vi "VI Tree - string__ogtk.vi"   [LabVIEW 2009]
uses:
  Trim Whitespace (String)__ogtk.vi
  Convert EOLs (String)__ogtk.vi
  To Camel Case (String)__ogtk.vi
  To Proper Case (String)__ogtk.vi
  To Proper Case (String Array)__ogtk.vi
  Trim Whitespace (String Array)__ogtk.vi
  To Camel Case (String Array)__ogtk.vi
  Convert EOLs (String Array)__ogtk.vi
panel:
  # "[OpenG VI Tags] ***Do Not Remove***"
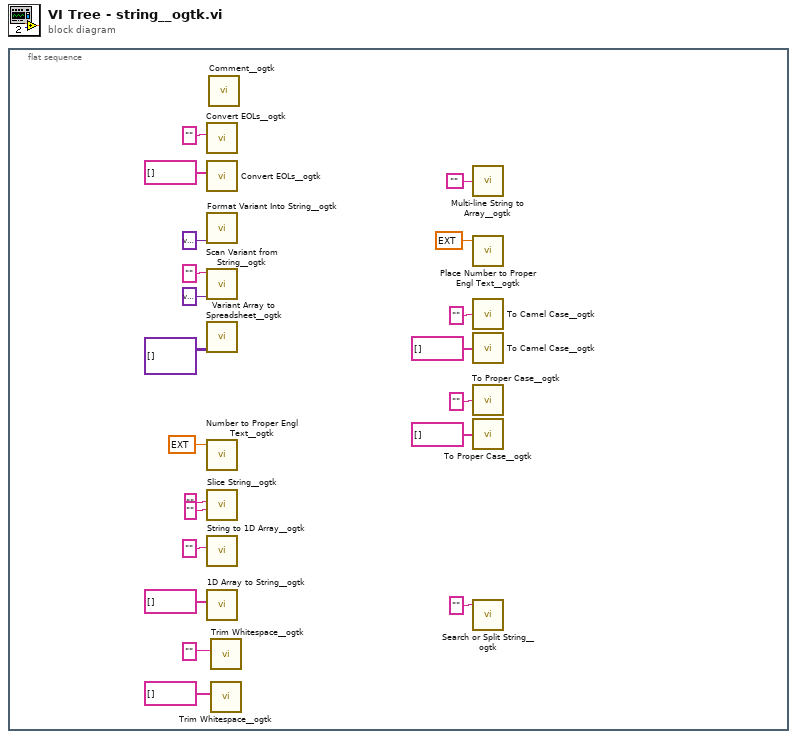
[diagram p0: block diagram]
diagram:
  n1 = flat-sequence {
    frame #0 {
      (unwired) "" ("string")
      n2 = call-poly "Convert EOLs__ogtk.vi"("String in"="") -> ()  [unwired: 10 in, 1 out]
      n3 = call-poly "Convert EOLs__ogtk.vi"("String in"=string[] [] ("strings")) -> ()  [unwired: 10 in, 1 out]
      n4 = call "Format Variant Into String__ogtk.vi"("Variant"=variant) -> ()  [unwired: 13 in, 2 out]
      n5 = call "Scan Variant from String__ogtk.vi"("Default Value"=variant, "Input String"="") -> ()  [unwired: 6 in, 4 out]
      n6 = call "Variant Array to Spreadsheet__ogtk.vi"("2D Variant Array"=variant[][] []) -> ()  [unwired: 9 in, 2 out]
      n7 = call "Number to Proper Engl Text__ogtk.vi"("Numeric"=ext 0.0) -> ()  [unwired: 4 in, 1 out]
      n8 = call "Slice String__ogtk.vi"("slice"="", "string"="") -> ()  [unwired: 5 in, 1 out]
      n9 = call "String to 1D Array__ogtk.vi"("string"="") -> ()  [unwired: 10 in, 1 out]
      n10 = call "1D Array to String__ogtk.vi"("Array of Strings"=string[] []) -> ()  [unwired: 10 in, 1 out]
      n11 = call "Comment__ogtk.vi"() -> ()  [unwired: 1 in]
      n12 = call-poly "Trim Whitespace__ogtk.vi"("String in"="") -> ()  [unwired: 6 in, 1 out]
      n13 = call-poly "Trim Whitespace__ogtk.vi"("String in"=string[] [] ("strings")) -> ()  [unwired: 6 in, 1 out]
      n14 = call "Multi-line String to Array__ogtk.vi"("string"="") -> ()  [unwired: 1 out]
      n15 = call "Place Number to Proper Engl Text__ogtk.vi"("Numeric"=ext 0.0) -> ()  [unwired: 4 in, 1 out]
      n16 = call-poly "To Camel Case__ogtk.vi"("string"="") -> ()  [unwired: 1 in, 1 out]
      n17 = call-poly "To Camel Case__ogtk.vi"("strings"=string[] []) -> ()  [unwired: 1 in, 1 out]
      n18 = call-poly "To Proper Case__ogtk.vi"("string"="") -> ()  [unwired: 4 in, 1 out]
      n19 = call-poly "To Proper Case__ogtk.vi"("strings"=string[] []) -> ()  [unwired: 4 in, 1 out]
      n20 = call "Search or Split String__ogtk.vi"("string"="") -> ()  [unwired: 2 in, 3 out]
    }
  }
